vi "all sensor graphbuffer.vi"(8 "Reset":bool, 9 "history length":u16=1000, 10 "WFGraph Refnum":refnum<vi>, 11 "Sensor Data":T1 {"Sensor array"."scaled" format="%.2f"; "Sensor array"."voltage" format="%.4f"; "Time" format="%<%I:%M:%S%2u %p\n%m/%d/%Y>T"}) -> (1 "data rate (Hz)":dbl format="%.2f", 2 "Mean":dbl[](array[numeric]) format="%.2f", 3 "Multiplot graph data":cluster{dbl[], dbl[]}[](array[cluster]) {"?" format="%.2f"; "?" format="%.2f"})   [LabVIEW 2015]
doc: "Takes an array containing one data point per channel and an arbitrary time. Creates data format required for an x-y plot with arbitrary data interval. Stores up to history number of data points per channel in a shift register.\nThis VI is reentrant meaning that it will hold different values if it is used at different places in a program. Thus more than one graph can be created!"
uses:
  TCP DAQ/Sensor data.ctl
  DAQ configuration/sensor cluster.ctl
  DAQ configuration/Sensor buffer command.ctl
  <vilib>/Analysis/baseanly.llb/Mean (DBL).vi
  <vilib>/Analysis/NI_AALBase.lvlib
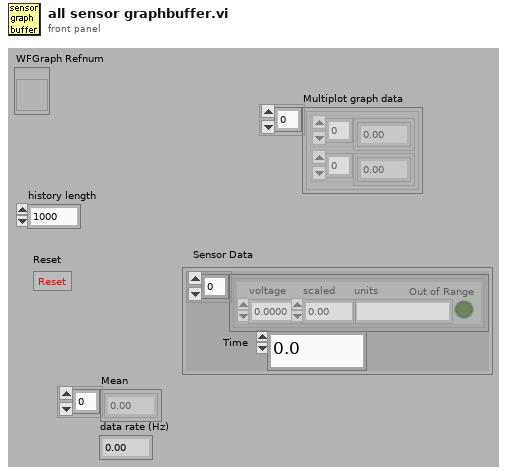
[diagram p1: front panel]
types:
  T1 = typedef "Sensor data.ctl" = cluster{" Sensor array":T2[], "Time":dbl}
  T2 = typedef "sensor cluster.ctl" = cluster{"voltage":sgl, "scaled":sgl, "units":string, "Out of Range":bool}
  T3 = typedef "Sensor buffer command.ctl" = enum16{"read average", "read recent", "read all", "write", "set buffer size", "Read channel config", "Write channel config", "clear"}
  T4 = typedef "Channel config.ctl" = cluster{"Channel Indices":T5[], "AI Max voltage":dbl[], "Calibration matrix":T6}
  T5 = typedef "channel identifier.ctl" = u16
  T6 = typedef "calib array.ctl" = T7[]
  T7 = typedef "conversion.ctl" = cluster{"conversion matrix":sgl[][], "units":string, "name":string, "scale type":T8, "offset (volts)":dbl, "second channel":i8, "correspondence table":T9, "offset (physical units)":dbl, "pH scale":T10, "D.O.":T11, "Photometer data":T12}
  T8 = typedef "scale type.ctl" = enum16{"Volts", "Polynomial", "Correspondence Table", "pH", "Dissolved Oxygen", "Quadratic", "Photometer"}
  T9 = typedef "correspondence table.ctl" = cluster{"physical units":dbl, "volts":dbl}[]
  T10 = typedef "pH scale.ctl" = cluster{"Buffers":cluster{"Buffer":dbl, "Calibrated":bool, "V/T":dbl}[], "Temperature":dbl}
  T11 = typedef "DO scale.ctl" = cluster{"Temperature":dbl, "K":dbl, "barometric pressure":dbl}
  T12 = typedef "Photometer calibration data.ctl" = cluster{"Dark Voltage":dbl, "Blank Voltage":dbl, "Standards":cluster{"Concentration":dbl, "Voltage":dbl}[]}
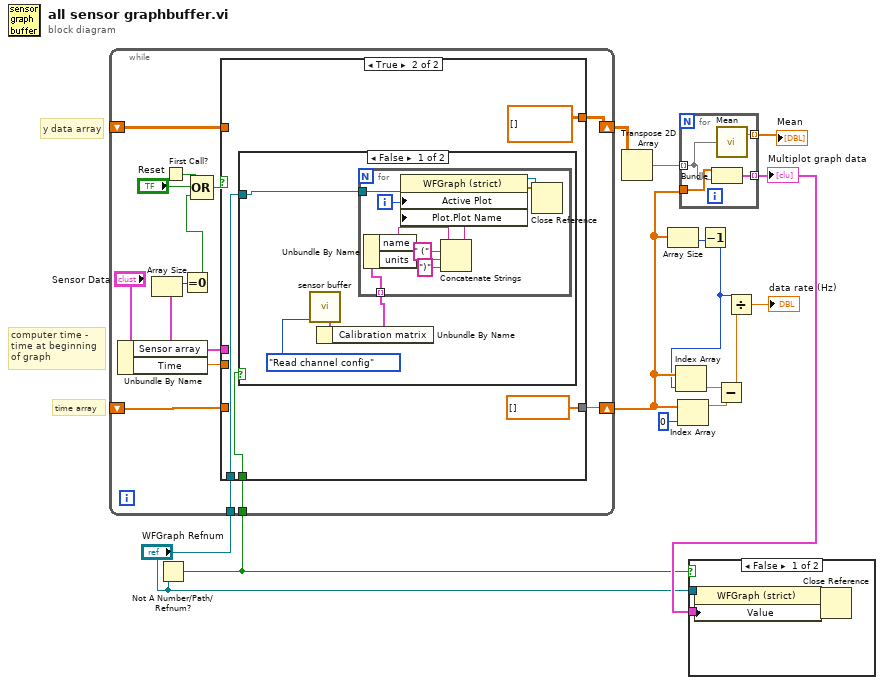
[diagram p0: block diagram]
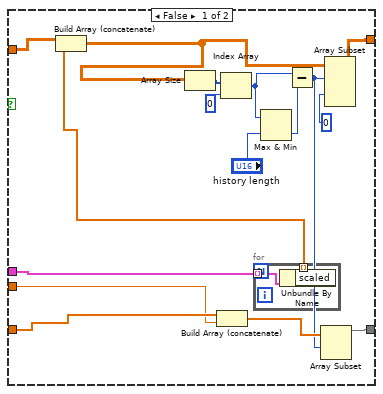
[diagram p3: hidden frame]
diagram:
  # "time array"
  # "y data array"
  # "computer time -  time at beginning of graph"
  n1 = Not A Number/Path/Refnum?(number/path/refnum="WFGraph Refnum") -> (NaN/Path/Refnum?=w1:bool)
  n2 = while {
    shift-left: _ -> [w27]
    shift-right: [w17] -> w10
    shift-left: _ -> [w29]
    shift-right: [w18] -> w14
    tunnel: "WFGraph Refnum" -> [w24]
    tunnel: w1 -> [w23]
    stop <- FALSE continue-if-true
    n3 = Unbundle By Name("Sensor Data") -> ("Sensor array"=w16:T2[], "Time"=w15:dbl)
    n4 = Array Size(array=w16) -> (size(s)=w20:i32)
    n5 = First Call?() -> (First Call?: T/F=w22:bool)
    n6 = Equal To 0?(x=w20) -> (x = 0?=w19:bool)
    n7 = Compound Arithmetic op=OR(w22, "Reset", w19) -> (w21:bool)
    n8 = case shown="True" w21 {
      tunnel: [w31 dbl[][] [] ("t")] -> w18
      tunnel: w29 -> [w35 _]
      tunnel: w27 -> [w34 _]
      tunnel: [w30 dbl[] []] -> w17
      tunnel: w24 -> [_ w49]
      tunnel: w23 -> [_ w48]
      tunnel: w16 -> [w33 _]
      tunnel: w15 -> [w32 _]
      frame False {
        n9 = Build Array (concatenate)(w34, w32) -> (w44:dbl[])
        n10 = for {
          tunnel: w33 -> [w47] mode=indexing
          tunnel: [w46] -> w45 mode=indexing
          n11 = Unbundle By Name(w47) -> ("scaled"=w46:sgl)
        }
        n12 = Build Array (concatenate)(w35, w45) -> (w36:dbl[][])
        n13 = Array Size(array=w36) -> (size(s)=w37:i32[])
        n14 = Index Array(array=w37, index=0 ("Index")) -> (element=w41:i32)
        n15 = Max & Min(x=w41, y="history length") -> (min(x,y)=w42:i32)  [unwired: 1 out]
        n16 = Subtract(x=w41, y=w42) -> (x-y=w43:i32)
        n17 = Array Subset(array=w44, index=w43) -> (w30:dbl[])  [unwired: 1 in]
        n18 = Array Subset(array=w36, index (row)=w43, index (col)=0 ("Array Index")) -> (w31:dbl[][])  [unwired: 2 in]
      }
      frame True {
        n19 = case shown="False" w48 {
          tunnel: w49 -> [w55 _]
          frame False {
            n20 = call "sensor buffer.vi"("command"=Sensor_buffer_command."Read channel config") -> ("Channel Config out"=w54:T4)  [unwired: 6 in, 4 out]
            n21 = Unbundle By Name(w54) -> ("Calibration matrix"=w52:T6)
            n22 = for {
              tunnel: w55 -> [w65]
              tunnel: w52 -> [w61] mode=indexing
              i -> [w64]
              n23 = Unbundle By Name(w61) -> ("name"=w60:string, "units"=w59:string)
              n24 = Concatenate Strings(w60, " (" ("string"), w59, ")" ("string")) -> (w56:string)
              n25 = property on="Property Node" class="WFGraph (strict)"(reference=w65, "Active Plot"=w64, "Plot.Plot Name"=w56) -> (reference out=w63:refnum<vi>, error out=w62:errorcluster)  [unwired: 1 in]
              n26 = Close Reference(reference=w63, error in (no error)=w62) -> ()  [unwired: 1 out]
            }
          }
          frame True {
          }
        }
      }
    }
  }
  n27 = Transpose 2D Array(2D array=w14) -> (transposed array=w12:dbl[][])
  n28 = Array Size(array=w10) -> (size(s)=w4:i32)
  n29 = Index Array(array=w10, index=0 ("Index")) -> (element=w7:dbl)
  n30 = for {
    tunnel: w12 -> [w67] mode=indexing
    tunnel: w10 -> [w69]
    tunnel: [w68] -> w13 mode=indexing
    tunnel: [w66] -> w11 mode=indexing
    n31 = Bundle(w69, w67) -> (w68:cluster{dbl[], dbl[]})  [unwired: 1 in]
    n32 = call-poly <vilib>:"Mean.vi"("X"=w67) -> ("mean"=w66:dbl)  [unwired: 1 out]
  }
  "Multiplot graph data" <- w13
  "Mean" <- w11
  n33 = case shown="False" w1 {
    tunnel: w13 -> [w73 _]
    tunnel: "WFGraph Refnum" -> [w70 _]
    frame False {
      n34 = property class="WFGraph (strict)"(reference=w70, "Value"=w73) -> (reference out=w71:refnum<vi>, error out=w72:errorcluster)  [unwired: 1 in]
      n35 = Close Reference(reference=w71, error in (no error)=w72) -> ()  [unwired: 1 out]
    }
    frame True {
    }
  }
  n36 = Decrement(x=w4) -> (x-1=w3:i32)
  n37 = Index Array(array=w10, index=w3) -> (element=w8:dbl)
  n38 = Subtract(x=w8, y=w7) -> (x-y=w6:dbl)
  n39 = Divide(x=w3, y=w6) -> (x/y=→"data rate (Hz)":dbl)
